vi "Write Configuration.vi"(8 "error in (no error)":errorcluster, 10 "Configuration":T1, 11 "ADAS PE Template in":refnum<class "ADAS PE Template.lvclass">) -> (0 "error out":errorcluster, 2 "Configure and Synchronize Required":bool, 3 "ADAS PE Template out":refnum<class "ADAS PE Template.lvclass">)   [LabVIEW 2020, in "ADAS PE Template.lvlib" / "ADAS PE Template.lvclass"]
doc: "<b>Write Configuration</b>\nBy default just store specified configuration and signal the PE state machine to reconfigure the PE"
uses:
  ADAS PE Template.lvclass
  Configuration.ctl
  ADAS PE Template.lvclass/ADAS PE Template.ctl
panel:
  # "#via_ignore"
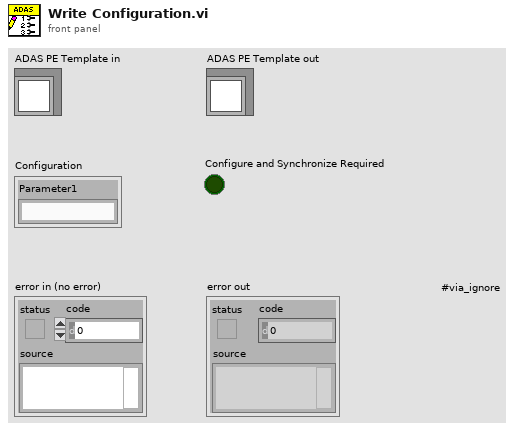
[diagram p1: front panel]
types:
  T1 = typedef "ADAS PE Template.lvlib/ADAS PE Template.lvclass/Configuration.ctl" = cluster{"Parameter1":string}
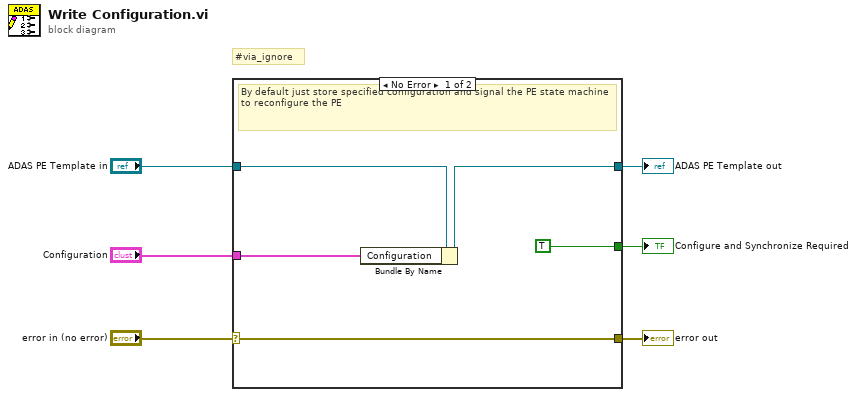
[diagram p0: block diagram]
diagram:
  # "#via_ignore"
  n1 = case shown="No Error" "error in (no error)" {
    selector: "error in (no error)" -> [w11 w12]
    tunnel: [w11 w12] -> w5
    tunnel: [w9 w13] -> w3
    tunnel: "ADAS PE Template in" -> [w10 w13]
    tunnel: "Configuration" -> [w8 _]
    tunnel: [TRUE ("Configure and Synchronize Required") _] -> w1
    frame No Error {
      # "By default just store specified configuration and signal the PE state machine to reconfigure the PE"
      n2 = Bundle By Name(cluster=w10, "Configuration"=w8) -> (w9:refnum<class "ADAS PE Template.lvclass">)
    }
    frame Error {
    }
  }
  "error out" <- w5
  "ADAS PE Template out" <- w3
  "Configure and Synchronize Required" <- w1
